vi "RNN - Save Params.vi"(0 "Parent Directory":path=path "C:/misc/LabVIEW/FILES", 1 "Child Directory":path=path "PARAMS/OUT", 2 "identifier":string="trial01~000", 4 "_params":T2={"Wxh"=[[0.08816814, 0.04683124, 0.055777, 0.09227439, -0.01918909, -0.07028967, 0.05425625, -0.0379505, 0.07987346, 0.0356478, 0.05973336, 0.16619236, 0.02046398, 0.09932278, -0.09221171, 0.05325043, -0.00535485, 0.03246301, -0.17515997, 0.03110044, 0.05437734, -0.16500322, 0.12000096, 0.1649645, 0.1031997, 2.2831364954098454, -0.26762318, 0.0756094, 0.18995645, 0.04524904, -0.00081326, -0.04883711, -0.14755549, -0.19723311, -0.00519835, 0.19983998, -0.14245144, 0.01749342, 0.10951843, 0.18386832, -0.06128515, 0.02890502, -0.026863, 0.07017105, -0.07696348, 0.08738502, 0.01626162, 0.01591019, -0.05762368, -0.02653832, -0.11843184, 0.07486549, -0.05592851, 0.05187977, -0.04329546, -0.6496044560076473, -0.07855285, 0.21604187, 0.17664132, 0.10618676, 0.05611695, 0.15389204, -0.0545733, -0.15482719, 0.07738559, 0.13691329, 0.0226289, 0.09086791, -0.03779128, 0.00199312, 0.04589986, 0.10173343, 0.0310035, -6.601754153091633, 0.18265082, 0.12041025, -0.1651582, -0.13558537, 0.02204783, -0.12710137, -0.10795069, -0.02992237, -0.00566535, -0.06157069, -0.07109834, -0.00666483, 0.20390881, 0.02221857, -0.04415688, 0.06551994, 7.126122830583855, -0.09587377, 0.17710312, -0.15125948, -0.05560332, -0.11110929, 0.06494723, -0.13095039, 0.0263675, -0.02231497], [-0.08343188, 0.13169153, 0.1288631, 0.0546262, -0.01746312, 0.06801226, -0.06002741, 0.05444902, -0.05028338, -0.03371919, 0.00843029, 0.0467597, -0.05651373, 0.20180604, -0.03855516, -0.04902326, 0.14263693, -0.04526089, 0.1481224, -0.08563165, -0.01876959, -0.24257298, 0.00668417, 0.04437711, -0.08505597, -4.751049856463012, -0.10709821, -0.08538787, 0.1252753, -0.01464419, 0.12482812, -0.0209396, 0.03716865, 0.05664404, 0.0996426, -0.08773137, 0.0559559, 0.17070887, -0.08276855, -0.1435454, 0.07794281, -0.06609533, 0.06617192, 0.04581866, -0.13316068, -0.02745144, -0.0805398, -0.04649653, 0.06018116, 0.0854968, -0.0708219, -0.08793426, 0.03763314, -0.1959806, 0.06112885, -5.935352511069194, -0.14912734, -0.04373468, -0.11244284, -0.05554647, -0.01623299, -0.13809015, 0.04418333, -0.06195049, -0.02999514, -0.08718573, 0.12812414, 0.14652069, 0.05450026, 0.08743315, -0.11138041, 0.09198846, 0.00600774, 3.387561522573733, -0.11309879, 0.05246258, -0.06254744, -0.1488877, 0.07818396, 0.14037968, 0.06683759, 0.06795294, -0.27167893, -0.03701823, -0.092279, 0.13621127, 0.09336218, 0.32174476, 0.03515643, -0.07317651, 5.189537892977786, -0.01430133, 0.30560519, -0.01141218, 0.04862607, -0.02174897, 0.07030534, -0.18104724, 0.07917192, 0.05820701]], "Whh"=[[1.4731669378116283, -6.396857932756678], [8.470540866165699, 0.9613814016230289]], "bh"=[[2.1751276593735414], [0.931608720011875]], "Why"=[[-2.45658257869901, -2.9773319925354618], [-2.5604218648870694, -3.09473551167835], [-2.565990190851571, -3.0608666391843884], [-2.551946695139124, -3.082348209362891], [-2.552612533435151, -3.071237976080961], [-2.5657379890846643, -3.068262765309522], [-2.559816550003393, -3.0624495678040606], [-2.542632685326276, -3.108659294034892], [-2.5578498891139074, -3.06753957854261], [-2.552103852801792, -3.0770341694988255], [-2.5492086926507618, -3.0930726907335684], [-2.5582061492700783, -3.072426374372152], [-2.5574130225392873, -3.051321742989122], [-2.5349635380291837, -3.0847967544987243], [-2.5597484977323868, -3.067344949585785], [-2.559331719436401, -3.0808369712324137], [-2.560417140348505, -3.067871919494536], [-2.5497421211595626, -3.099703507049692], [-2.564397973697664, -3.0655683595821808], [-2.5525709975619306, -3.055900939601543], [-2.560166771612232, -3.042262375133108], [-2.5501632868769892, -3.0649873911183283], [-2.5713303530719247, -3.0847914453578307], [-2.5722867059735037, -3.058501456536748], [-2.563584676293062, -3.0525342346877617], [10.937254918668582, 2.4693802865943977], [-2.560099661343097, -3.0655683787759322], [-2.549948454944238, -3.1057541409099354], [-2.545166182401163, -3.1070126919928818], [-2.5553920072175234, -3.082746301141685], [-2.5718860479636736, -3.045545705860628], [-2.538768941369366, -3.0597366208275703], [-2.5657915198170227, -3.045500982927337], [-2.563587499863479, -3.0996356811378467], [-2.572910718383849, -3.084733048541443], [-2.556007192877619, -3.075185758449212], [-2.5568973980152156, -3.041214221272187], [-2.5489224053202917, -3.100511898478674], [-2.542046048209207, -3.083421721421329], [-2.5495721896870047, -3.0643573252154463], [-2.5564996466915195, -3.069422601232006], [-2.550986016407652, -3.066351988471276], [-2.5595004063047613, -3.0824342525647723], [-2.567779642791458, -3.042810969455463], [-2.543171536360651, -3.083662936329873], [-2.566309282592417, -3.114066150391768], [-2.5427207567948624, -3.0472618984559774], [-2.560526338221769, -3.096029845912513], [-2.568945626882554, -3.0775875663784853], [-2.56058161285034, -3.0887516330860008], [-2.567989573900908, -3.07759009916362], [-2.5452228209567993, -3.0685195926378683], [-2.556067764597753, -3.088477889327711], [-2.5378840375795897, -3.063808658036209], [-2.570184171626281, -3.0653089331888648], [-7.292051927025788, 3.3235427506251995], [-2.5643026259284607, -3.1001331375874552], [-2.5459227853924387, -3.0815245169020136], [-2.5523684671913944, -3.0920053289330136], [-2.54977248000111, -3.06521877980227], [-2.5426195643899963, -3.0705020361496893], [-2.543729505880343, -3.058644451384166], [-2.5466804114677424, -3.089091538476544], [-2.54590545725718, -3.0650949300275068], [-2.5545900748072765, -3.098678797259642], [-2.5333413557514097, -3.075066391586879], [-2.54766114761315, -3.123629596037064], [-2.541804407434486, -3.074912269478546], [-2.548183544898893, -3.0577019175518845], [-2.564863666773275, -3.0581414570487464], [-2.551476740733705, -3.0956569648936636], [-2.558929784054938, -3.063971188458965], [-2.5478837615534666, -3.081731169996417], [-14.289369111180172, -7.4885478825935285], [-2.565148348714134, -3.0791250954650575], [-2.552587464527017, -3.0513997083500812], [-2.554589638779874, -3.1036182903908616], [-2.5477690950446905, -3.078625811560547], [-2.54461411921147, -3.0605290798937954], [-2.574662373517977, -3.0814339433473728], [-2.5741055348058905, -3.070147902660904], [-2.557515059203827, -3.0593259184843222], [-2.5423498393037325, -3.0945708168633352], [-2.553627206306344, -3.091376228511211], [-2.54088111609538, -3.0558889583310798], [-2.5700828266221154, -3.086918193728097], [-2.5628843866599857, -3.0753264138404632], [-2.544507262143471, -3.0347170905804197], [-2.551781324149966, -3.067833183694833], [-2.535147873906761, -3.0889324100089435], [4.050940417334607, -8.530936407804598], [-2.5514157919234117, -3.070061535732613], [-2.5641915601746774, -3.099881878621316], [-2.571557819356872, -3.0485518191580536], [-2.5478333964918325, -3.034415373942667], [-2.5533264939186195, -3.0690790936514047], [-2.5372156597997058, -3.0774939371757317], [-2.5658895986641155, -3.1023237744346637], [-2.5671532924444214, -3.0858629120703784], [-2.569702622109911, -3.0490610923870753]], "by"=[[-9.6939417702583], [-9.787461452991378], [-9.795880424049155], [-9.791754680172033], [-9.795466938501924], [-9.792349266631804], [-9.799776783437428], [-9.786104428615676], [-9.795907459503352], [-9.795268706938119], [-9.789698172547547], [-9.794336448453244], [-9.800008814538856], [-9.795556283704723], [-9.79501577752053], [-9.794266275161212], [-9.794349322608694], [-9.788410913635246], [-9.795723007815635], [-9.802258680652661], [-9.802432856674923], [-9.798080755131593], [-9.78834097315508], [-9.7946552477736], [-9.799128361260347], [-5.0269669804907995], [-9.793598741934135], [-9.784613485603533], [-9.78646503211266], [-9.792353819871323], [-9.803918973327148], [-9.80248199928148], [-9.800975798298028], [-9.785919285886518], [-9.787967678198404], [-9.792189683909982], [-9.803416273020147], [-9.785399189075022], [-9.792344159342278], [-9.799759065599373], [-9.795434869135798], [-9.798104867799251], [-9.79098036886028], [-9.80181961852864], [-9.79247681843316], [-9.778943227920282], [-9.804318999722339], [-9.786169938427546], [-9.7917473961263], [-9.787472191742584], [-9.793264780681755], [-9.796822458370732], [-9.789871238562121], [-9.799613902468865], [-9.794489448255803], [0.053253287043484795], [-9.784803341418362], [-9.795027557753857], [-9.788939930062503], [-9.79758559829949], [-9.798039859067053], [-9.80192835313501], [-9.791961705041455], [-9.796892314417502], [-9.785892415386455], [-9.797135901569282], [-9.781318785731925], [-9.796595812788555], [-9.802023321961775], [-9.799158831982991], [-9.787294065481879], [-9.79712631429669], [-9.791608695796691], [-4.671542944905596], [-9.79261449202089], [-9.80180477179711], [-9.786181349062877], [-9.792118485010652], [-9.797477226045931], [-9.78955617652576], [-9.793088478557278], [-9.797484028737504], [-9.787503430892013], [-9.789925704374266], [-9.799513676082261], [-9.787678112179325], [-9.793571042223654], [-9.80880382890866], [-9.79650163017262], [-9.79252806896738], [-0.19883449486869695], [-9.79305207299255], [-9.785793938857388], [-9.798245019409398], [-9.807212051036144], [-9.79690305644076], [-9.795699835304656], [-9.785360495953634], [-9.786913136541566], [-9.802458269440217]]}) -> (15 "Saved":bool, 18 "Paths":path[](array[path])=[path "C:/misc/LabVIEW/FILES/PARAMS/OUT/Wxh_trial01.psv", path "C:/misc/LabVIEW/FILES/PARAMS/OUT/Whh_trial01.psv", path "C:/misc/LabVIEW/FILES/PARAMS/OUT/bh_trial01.psv", path "C:/misc/LabVIEW/FILES/PARAMS/OUT/Why_trial01.psv", path "C:/misc/LabVIEW/FILES/PARAMS/OUT/by_trial01.psv"])   [LabVIEW 2014]
uses:
  <vilib>/Analysis/Matrix/Datatypes/RealMatrix.ctl
  <vilib>/Analysis/Matrix/NI_Matrix.lvlib
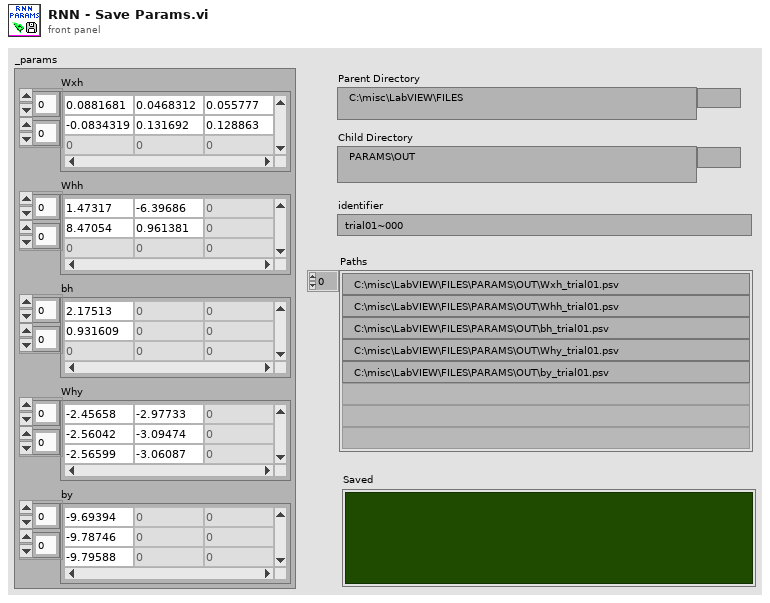
[diagram p1: front panel]
types:
  T1 = typedef "NI_Matrix.lvlib/RealMatrix.ctl" = dbl[][]
  T2 = cluster{"Wxh":T1, "Whh":T1, "bh":T1, "Why":T1, "by":T1}
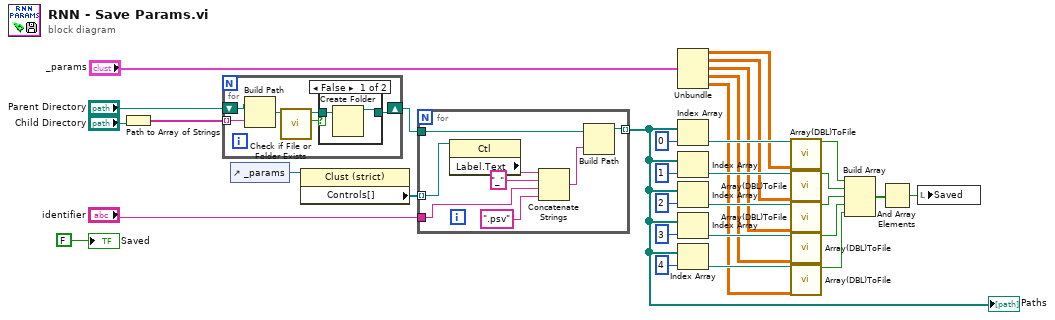
[diagram p0: block diagram]
diagram:
  n1 = Path to Array of Strings(0:"Child Directory") -> (2:w3:string[])  [unwired: 1 out]
  n2 = for {
    tunnel: w3 -> [w37] mode=indexing
    shift-right: [w33] -> w1
    shift-left: "Parent Directory" -> [w38]
    n3 = Build Path(base path=w38, name or relative path=w37) -> (appended path=w36:path)
    n4 = call <vilib>:"Check if File or Folder Exists.vi"("path"=w36) -> ("file or folder exists?"=w35:bool, "dup path"=w34:path)  [unwired: 8 in, 1 out]
    n5 = case shown="False" w35 {
      tunnel: w34 -> [w40 w41]
      tunnel: [w39 w41] -> w33
      frame False {
        n6 = Create Folder(path (use dialog)=w40) -> (created path=w39:path)  [unwired: 2 in, 2 out]
      }
      frame True {
      }
    }
  }
  n7 = control-ref of="_params"() -> (w13:refnum<vi>)
  n8 = property class="Clust (strict)"(reference=w13) -> ("Controls[]"=w15:refnum<vi>[])  [unwired: 1 in, 2 out]
  n9 = for {
    tunnel: w15 -> [w45] mode=indexing
    tunnel: w1 -> [w49]
    tunnel: [w48] -> w32 mode=indexing
    tunnel: "identifier" -> [w42]
    n10 = property class="Ctl"(reference=w45) -> ("Label.Text"=w46:string)  [unwired: 1 in, 2 out]
    n11 = Concatenate Strings(w46, "_" ("string"), w42, ".psv" ("string")) -> (w47:string)
    n12 = Build Path(base path=w49, name or relative path=w47) -> (appended path=w48:path)
  }
  "Paths" <- w32
  n13 = Unbundle("_params") -> ("Wxh"=w14:T1, "Whh"=w18:T1, "bh"=w20:T1, "Why"=w21:T1, "by"=w22:T1)
  n14 = Index Array(array=w32, index=0) -> (element=w26:path)
  n15 = Index Array(array=w32, index=1) -> (element=w27:path)
  n16 = Index Array(array=w32, index=2) -> (element=w28:path)
  n17 = Index Array(array=w32, index=3) -> (element=w29:path)
  n18 = Index Array(array=w32, index=4) -> (element=w30:path)
  n19 = call "Array(DBL)ToFile.vi"("path"=w26, "Array(2D)"=w14) -> ("Saved"=w12:bool)  [unwired: 16 in, 1 out]
  n20 = call "Array(DBL)ToFile.vi"("path"=w27, "Array(2D)"=w18) -> ("Saved"=w11:bool)  [unwired: 16 in, 1 out]
  n21 = call "Array(DBL)ToFile.vi"("path"=w28, "Array(2D)"=w20) -> ("Saved"=w10:bool)  [unwired: 16 in, 1 out]
  n22 = call "Array(DBL)ToFile.vi"("path"=w29, "Array(2D)"=w21) -> ("Saved"=w9:bool)  [unwired: 16 in, 1 out]
  n23 = call "Array(DBL)ToFile.vi"("path"=w30, "Array(2D)"=w22) -> ("Saved"=w8:bool)  [unwired: 16 in, 1 out]
  n24 = Build Array(w12, w11, w10, w9, w8) -> (w7:bool[])
  n25 = And Array Elements(Boolean array=w7) -> (logical AND=w5:bool)
  n26 = local write "Saved"(w5) -> ()
  "Saved" <- FALSE
